vi "Open Report.vi"() -> ()   [LabVIEW 2016, in "Data Operations.lvlib"]
uses:
  Data Operations.lvlib
panel:
  in  "Data Value Refnum 2":refnum<data-value>
  out "data value":dbl
  out "Data Value Refnum":refnum<data-value>
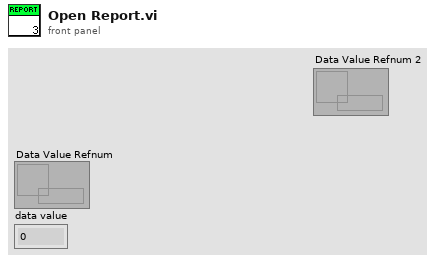
[diagram p1: front panel]
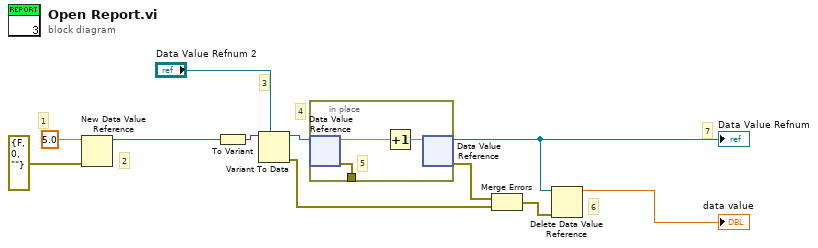
[diagram p0: block diagram]
diagram:
  # "7"
  # "6"
  # "4"
  # "3"
  # "2"
  # "1"
  n1 = New Data Value Reference(data value=5.0, error in=errorcluster {"status"=FALSE, "code"=0, "source"=""}) -> (data value reference=w10:refnum<data-value>)  [unwired: 1 out]
  n2 = To Variant(anything=w10) -> (Variant=w9:variant)
  n3 = Variant To Data(type="Data Value Refnum 2", Variant=w9) -> (data=w4:refnum<data-value>, error out=w3:errorcluster)  [unwired: 1 in]
  n4 = in-place "In Place Element Structure" {
    in-place-border: [w12] -> _
    # "5"
    n5 = in-place-dvr #1(w4) -> (w14:dbl, w12:errorcluster)
    n6 = Increment(x=w14) -> (x+1=w13:dbl)
    n7 = in-place-dvr #1(w13) -> (w7:refnum<data-value>, w2:errorcluster)
  }
  "Data Value Refnum" <- w7
  n8 = Merge Errors(w2, w3) -> (w1:errorcluster)
  n9 = Delete Data Value Reference(data value reference=w7, error in=w1) -> (data value=→"data value":dbl)  [unwired: 1 out]
